vi "DetermineNumberofPointsperPlane.vi"(8 "error in (no error)":errorcluster, 10 "DutyCluster":T1 {"Iteration" items=["first iteration", "second iteration"]}, 11 "XY coordinates (um)":dbl[][](array[numeric])) -> (0 "error out":errorcluster, 3 "DutyCluster":T1 {"Iteration" items=["first iteration", "second iteration"]})   [LabVIEW 2010]
uses:
  TypeDefs/DutyCluster.ctl
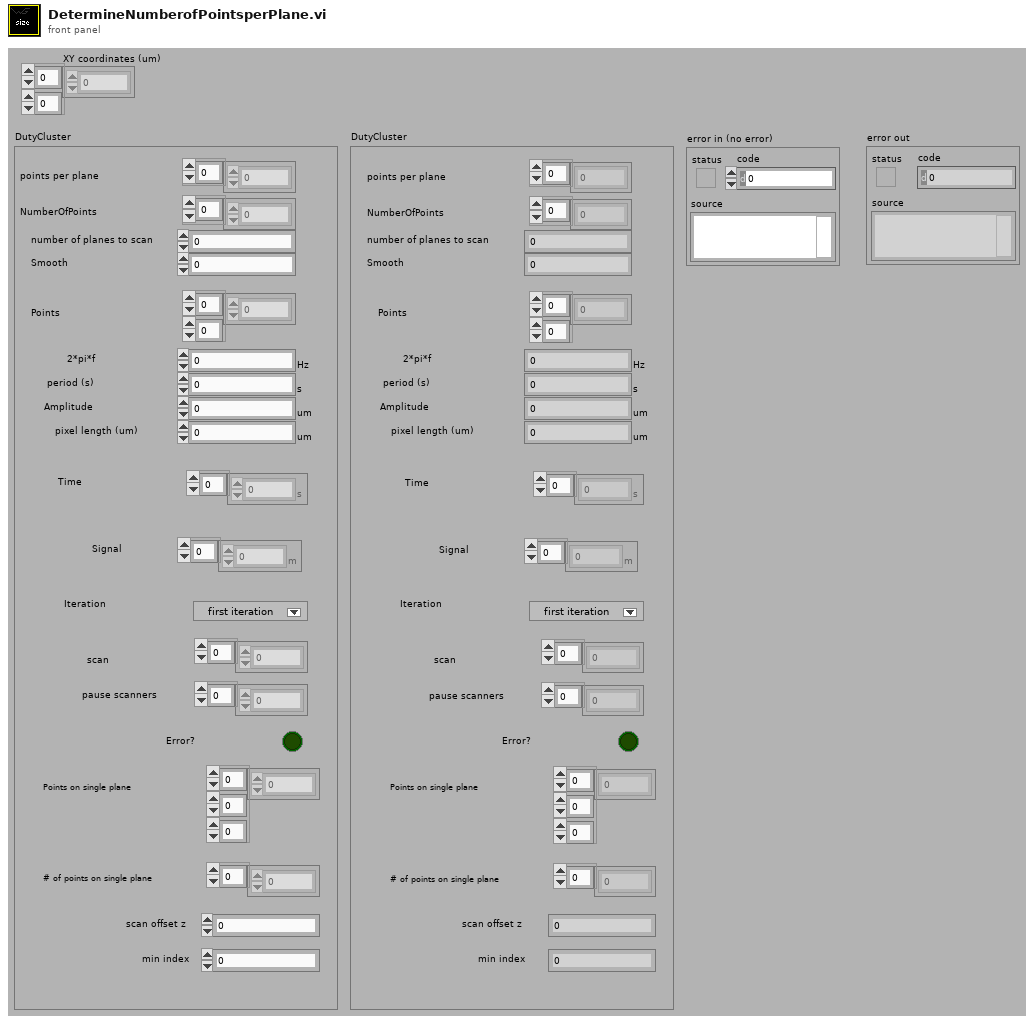
[diagram p1: front panel]
types:
  T1 = typedef "DutyCluster.ctl" = cluster{"points per plane":i32[], "NumberOfPoints":i32[], "number of planes to scan":i32, "Smooth":i32, "Points":dbl[][], "2*pi*f":dbl[unit], "period (s)":dbl[unit], "Amplitude":dbl[unit], "pixel length (um)":dbl[unit], "Time":dbl[unit][], "Signal":dbl[unit][], "Iteration":u16, "scan":i32[], "pause scanners":i32[], "Error?":bool, "Points on single plane":dbl[][][], "# of points on single plane":i32[], "scan offset z":i32, "min index":i32}
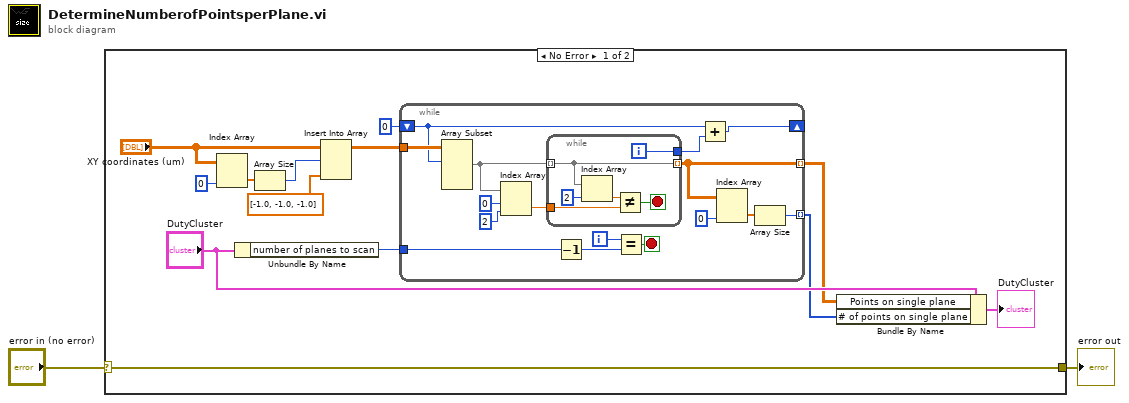
[diagram p0: block diagram]
diagram:
  n1 = case shown="No Error" "error in (no error)" {
    selector: "error in (no error)" -> [w3 w38]
    tunnel: [w3 w38] -> w1
    frame No Error {
      n2 = Index Array(array="XY coordinates (um)", index (col)=0 ("disabled index (col)")) -> (element=w12:dbl[])  [unwired: 1 in]
      n3 = Unbundle By Name("DutyCluster") -> ("number of planes to scan"=w9:i32)
      n4 = Array Size(array=w12) -> (size(s)=w11:i32)
      n5 = Insert Into Array(array="XY coordinates (um)", index (row)=w11, new element=dbl[] [-1.0, -1.0, -1.0] ("new element/subarray")) -> (w10:dbl[][])  [unwired: 1 in]
      n6 = while {
        tunnel: w10 -> [w30]
        shift-right: [w31] -> _
        shift-left: 0 -> [w26]
        tunnel: [w18] -> w5 mode=indexing
        tunnel: w9 -> [w24]
        tunnel: [w17] -> w6 mode=indexing
        i -> [w29]
        stop <- w28 stop-if-true
        n7 = Array Subset(array=w30, index (row)=w26) -> (w23:dbl[][])  [unwired: 3 in]
        n8 = Index Array(array=w23, index (row)=0 ("disabled index (row)"), index (col)=2 ("disabled index (col)")) -> (element=w25:dbl)
        n9 = while {
          tunnel: w23 -> [w35] mode=indexing
          tunnel: [w35] -> w18 mode=indexing
          tunnel: [w34] -> w19
          tunnel: w25 -> [w33]
          i -> [w34]
          stop <- w36 stop-if-true
          n10 = Index Array(array=w35, index=2) -> (element=w32:dbl)
          n11 = Not Equal?(x=w32, y=w33) -> (x != y?=w36:bool)
        }
        n12 = Decrement(x=w24) -> (x-1=w16:i32)
        n13 = Equal?(x=w29, y=w16) -> (x = y?=w28:bool)
        n14 = Add(x=w26, y=w19) -> (x+y=w31:i32)
        n15 = Index Array(array=w18, index (col)=0 ("disabled index (col)")) -> (element=w21:dbl[])  [unwired: 1 in]
        n16 = Array Size(array=w21) -> (size(s)=w17:i32)
      }
      n17 = Bundle By Name(cluster="DutyCluster", "Points on single plane"=w5, "# of points on single plane"=w6) -> (→"DutyCluster":T1)
    }
    frame Error {
    }
  }
  "error out" <- w1
